vi "Menu.vi"(7 "action":T1, 8 "error in":errorcluster, 10 "item tag":string, 11 "menu reference":refnum<k9>) -> (0 "error out":errorcluster, 1 "item index":i32, 2 "Item Present?":bool, 3 "item tag":string)   [LabVIEW 2011]
uses:
  Menu Action.ctl
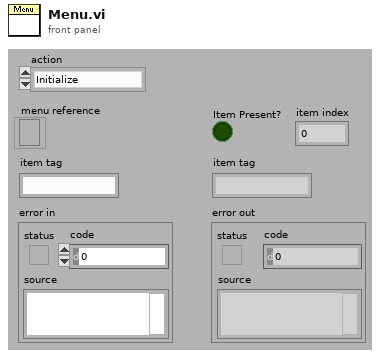
[diagram p1: front panel]
types:
  T1 = typedef "Menu Action.ctl" = enum16{"Initialize", "Insert Item", "Remove Item", "Set Checked Item", "Get Checked Item", "Get Item Index", "Item Present?", "Stop"}
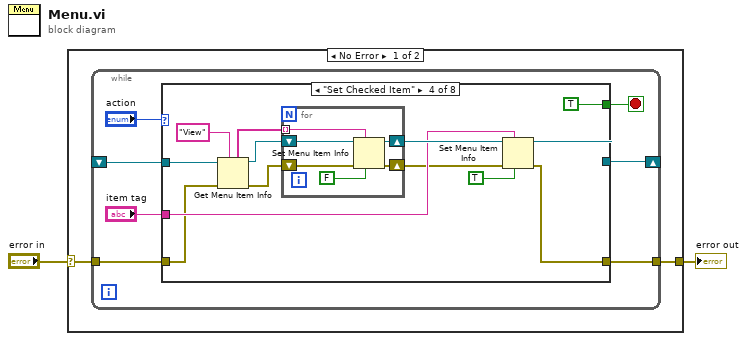
[diagram p0: block diagram]
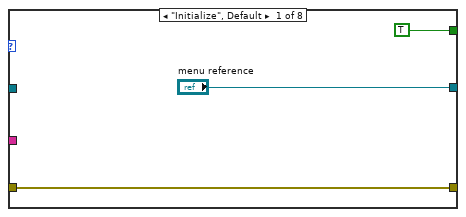
[diagram p2: hidden frame]
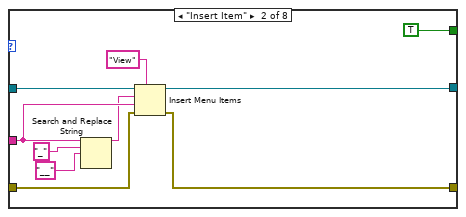
[diagram p3: hidden frame]
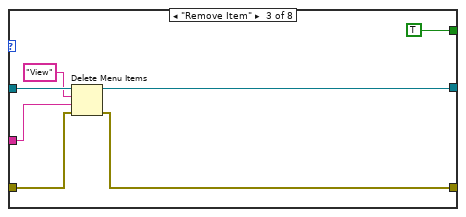
[diagram p4: hidden frame]
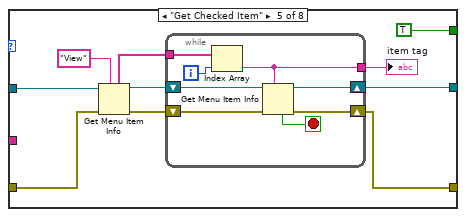
[diagram p5: hidden frame]
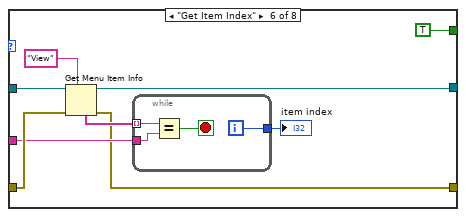
[diagram p6: hidden frame]
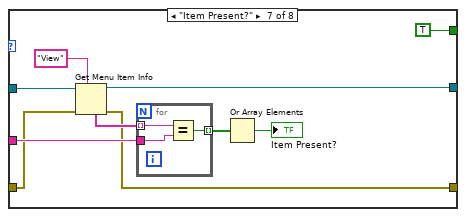
[diagram p7: hidden frame]
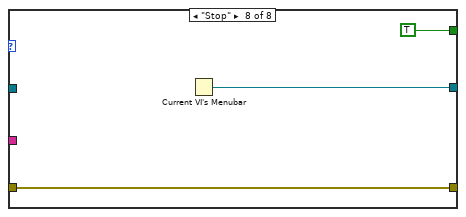
[diagram p8: hidden frame]
diagram:
  n1 = case shown="No Error" "error in" {
    selector: "error in" -> [w4 w98]
    tunnel: [w3 w98] -> w1
    frame No Error {
      n2 = while {
        tunnel: w4 -> [w11]
        tunnel: [w10] -> w3
        shift-right: [w9] -> _
        shift-left: _ -> [w8]
        stop <- w6 stop-if-true
        n3 = case shown="\"Set Checked Item\"" "action" {
          tunnel: w11 -> [w14 w16 w30 w37 w58 w75 w83 w96]
          tunnel: [w14 w15 w29 w34 w53 w71 w82 w96] -> w10
          tunnel: ["menu reference" w22 w28 w33 w52 w72 w86 w97] -> w9
          tunnel: w8 -> [_ w24 w31 w44 w60 w76 w90 _]
          tunnel: "item tag" -> [_ w20 w26 w39 _ w73 w87 _]
          tunnel: [TRUE TRUE TRUE TRUE TRUE TRUE TRUE TRUE] -> w6
          frame "Initialize", Default {
          }
          frame "Insert Item" {
            n4 = Search and Replace String(input string=w20, search string="_", replace string="__" ("replace string (\"\")")) -> (result string=w17:string)  [unwired: 5 in, 3 out]
            n5 = Insert Menu Items(5:"View" ("menu tag"), 6:w16, 7:w20, 8:w17, 9:w24) -> (0:w15:errorcluster, 3:w22:refnum<k9>)  [unwired: 1 in, 1 out]
          }
          frame "Remove Item" {
            n6 = Delete Menu Items(6:w30, 7:w26, 8:"View" ("menu tag"), 9:w31) -> (0:w29:errorcluster, 3:w28:refnum<k9>)
          }
          frame "Set Checked Item" {
            n7 = Get Menu Item Info(7:"View" ("item tag"), 8:w37, 11:w44) -> (0:w35:errorcluster, 3:w40:refnum<k9>, 5:w42:string[])  [unwired: 4 out]
            n8 = for {
              tunnel: w42 -> [w49] mode=indexing
              shift-right: [w47] -> w41
              shift-left: w40 -> [w50]
              shift-right: [w46] -> w36
              shift-left: w35 -> [w45]
              n9 = Set Menu Item Info(6:FALSE ("checked"), 7:w49, 8:w45, 11:w50) -> (0:w46:errorcluster, 3:w47:refnum<k9>)  [unwired: 3 in]
            }
            n10 = Set Menu Item Info(6:TRUE ("checked"), 7:w39, 8:w36, 11:w41) -> (0:w34:errorcluster, 3:w33:refnum<k9>)  [unwired: 3 in]
          }
          frame "Get Checked Item" {
            n11 = Get Menu Item Info(7:"View" ("item tag"), 8:w58, 11:w60) -> (0:w54:errorcluster, 3:w57:refnum<k9>, 5:w56:string[])  [unwired: 4 out]
            n12 = while {
              shift-right: [w67] -> w52
              shift-left: w57 -> [w68]
              tunnel: w56 -> [w65]
              tunnel: [w63] -> w55
              shift-right: [w61] -> w53
              shift-left: w54 -> [w62]
              i -> [w64]
              stop <- w66 stop-if-true
              n13 = Index Array(array=w65, index=w64) -> (element=w63:string)
              n14 = Get Menu Item Info(7:w63, 8:w62, 11:w68) -> (0:w61:errorcluster, 3:w67:refnum<k9>, 4:w66:bool)  [unwired: 4 out]
            }
            "item tag" <- w55
          }
          frame "Get Item Index" {
            n15 = Get Menu Item Info(7:"View" ("item tag"), 8:w75, 11:w76) -> (0:w71:errorcluster, 3:w72:refnum<k9>, 5:w74:string[])  [unwired: 4 out]
            n16 = while {
              tunnel: w74 -> [w81] mode=indexing
              tunnel: w73 -> [w80]
              tunnel: [w78] -> w70
              i -> [w78]
              stop <- w79 stop-if-true
              n17 = Equal?(x=w81, y=w80) -> (x = y?=w79:bool)
            }
            "item index" <- w70
          }
          frame "Item Present?" {
            n18 = Get Menu Item Info(7:"View" ("item tag"), 8:w83, 11:w90) -> (0:w82:errorcluster, 3:w86:refnum<k9>, 5:w88:string[])  [unwired: 4 out]
            n19 = for {
              tunnel: w88 -> [w94] mode=indexing
              tunnel: w87 -> [w93]
              tunnel: [w92] -> w85 mode=indexing
              n20 = Equal?(x=w94, y=w93) -> (x = y?=w92:bool)
            }
            n21 = Or Array Elements(Boolean array=w85) -> (logical OR=→"Item Present?":bool)
          }
          frame "Stop" {
            n22 = Current VI's Menubar() -> (w97:refnum<k9>)
          }
        }
      }
    }
    frame Error {
    }
  }
  "error out" <- w1
